vi "Write Rx Data Type.vi"(8 "error in (no error)":errorcluster, 10 "Data Type":T1, 11 "Node Ptr":T2 format="%.0x") -> (0 "error out":errorcluster, 3 "Node Ptr out":T2 format="%.0x")   [LabVIEW 2023, in "UDP-Custom-Device System Explorer.lvlib" / "Rx Channel Accessors.lvlib"]
uses:
  Rx Channel Accessors.lvlib
  <vilib>/NI VeriStand/Custom Device API/Custom Device Item Ref.ctl
  Shared/Types/Shared - Channel Data Type.ctl
  Shared/Constants.vi
  <vilib>/NI VeriStand/Custom Device API/Set Item Property (U16).vi
  <vilib>/NI VeriStand/Custom Device API/Custom Device API.lvlib
  Shared/UDP-Custom-Device Shared.lvlib
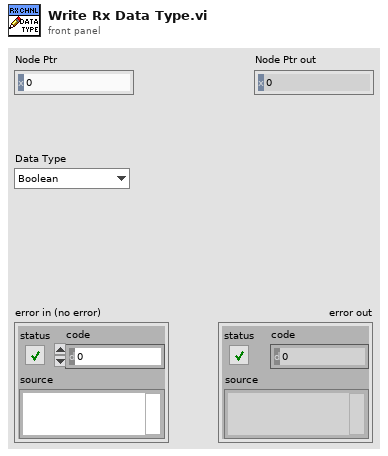
[diagram p1: front panel]
types:
  T1 = typedef "UDP-Custom-Device Shared.lvlib/Shared - Channel Data Type.ctl" = enum16{"Boolean", "Single", "Double", "I8", "I16", "I32", "I64", "U8", "U16", "U32", "U64"}
  T2 = typedef "Custom Device API.lvlib/Custom Device Item Ref.ctl" = u64
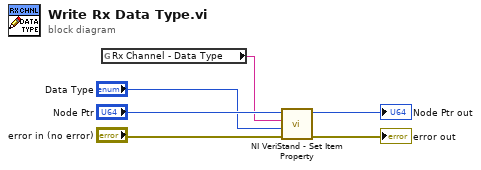
[diagram p0: block diagram]
diagram:
  n1 = global read "Constants.vi" "Rx Channel - Data Type"() -> (w1:string)
  n2 = call-poly <vilib>:"NI VeriStand - Set Item Property.vi"("error in (no error)"="error in (no error)", "Value"="Data Type", "Property Name"=w1, "Item Ref in"="Node Ptr") -> ("error out"=→"error out":errorcluster, "Item Ref out"=→"Node Ptr out":T2)  [unwired: 5 in, 1 out]
